vi "OCV Histogram gRPC.vi"() -> (1 "mean values of channels":dbl[](array[numeric]), 2 "std dev":dbl, 3 "range":dbl)   [LabVIEW 2019] (continued)
"battery23voltage"=0.0, "battery24voltage"=0.0, "ErrorOutData"={"ErrorCode"=0, "ErrorMessage"=""}}, {"battery1voltage"=3.48165, "battery2voltage"=3.4830537, "battery3voltage"=3.478374, "battery4voltage"=3.482381, "battery5voltage"=3.4844167, "battery6voltage"=0.0, "battery7voltage"=0.0, "battery8voltage"=0.0, "battery9voltage"=0.0, "battery10voltage"=0.0, "battery11voltage"=0.0, "battery12voltage"=0.0, "battery13voltage"=0.0, "battery14voltage"=0.0, "battery15voltage"=0.0, "battery16voltage"=0.0, "battery17voltage"=0.0, "battery18voltage"=0.0, "battery19voltage"=0.0, "battery20voltage"=0.0, "battery21voltage"=0.0, "battery22voltage"=0.0, "battery23voltage"=0.0, "battery24voltage"=0.0, "ErrorOutData"={"ErrorCode"=0, "ErrorMessage"=""}}, {"battery1voltage"=3.4816468, "battery2voltage"=3.4830554, "battery3voltage"=3.478373, "battery4voltage"=3.482378, "battery5voltage"=3.4844193, "battery6voltage"=0.0, "battery7voltage"=0.0, "battery8voltage"=0.0, "battery9voltage"=0.0, "battery10voltage"=0.0, "battery11voltage"=0.0, "battery12voltage"=0.0, "battery13voltage"=0.0, "battery14voltage"=0.0, "battery15voltage"=0.0, "battery16voltage"=0.0, "battery17voltage"=0.0, "battery18voltage"=0.0, "battery19voltage"=0.0, "battery20voltage"=0.0, "battery21voltage"=0.0, "battery22voltage"=0.0, "battery23voltage"=0.0, "battery24voltage"=0.0, "ErrorOutData"={"ErrorCode"=0, "ErrorMessage"=""}}, {"battery1voltage"=3.4816458, "battery2voltage"=3.4830527, "battery3voltage"=3.4783716, "battery4voltage"=3.4823792, "battery5voltage"=3.4844203, "battery6voltage"=0.0, "battery7voltage"=0.0, "battery8voltage"=0.0, "battery9voltage"=0.0, "battery10voltage"=0.0, "battery11voltage"=0.0, "battery12voltage"=0.0, "battery13voltage"=0.0, "battery14voltage"=0.0, "battery15voltage"=0.0, "battery16voltage"=0.0, "battery17voltage"=0.0, "battery18voltage"=0.0, "battery19voltage"=0.0, "battery20voltage"=0.0, "battery21voltage"=0.0, "battery22voltage"=0.0, "battery23voltage"=0.0, "battery24voltage"=0.0, "ErrorOutData"={"ErrorCode"=0, "ErrorMessage"=""}}, {"battery1voltage"=3.4816468, "battery2voltage"=3.4830546, "battery3voltage"=3.4783747, "battery4voltage"=3.4823809, "battery5voltage"=3.4844174, "battery6voltage"=0.0, "battery7voltage"=0.0, "battery8voltage"=0.0, "battery9voltage"=0.0, "battery10voltage"=0.0, "battery11voltage"=0.0, "battery12voltage"=0.0, "battery13voltage"=0.0, "battery14voltage"=0.0, "battery15voltage"=0.0, "battery16voltage"=0.0, "battery17voltage"=0.0, "battery18voltage"=0.0, "battery19voltage"=0.0, "battery20voltage"=0.0, "battery21voltage"=0.0, "battery22voltage"=0.0, "battery23voltage"=0.0, "battery24voltage"=0.0, "ErrorOutData"={"ErrorCode"=0, "ErrorMessage"=""}}, {"battery1voltage"=3.4816499, "battery2voltage"=3.483051, "battery3voltage"=3.4783742, "battery4voltage"=3.4823804, "battery5voltage"=3.4844172, "battery6voltage"=0.0, "battery7voltage"=0.0, "battery8voltage"=0.0, "battery9voltage"=0.0, "battery10voltage"=0.0, "battery11voltage"=0.0, "battery12voltage"=0.0, "battery13voltage"=0.0, "battery14voltage"=0.0, "battery15voltage"=0.0, "battery16voltage"=0.0, "battery17voltage"=0.0, "battery18voltage"=0.0, "battery19voltage"=0.0, "battery20voltage"=0.0, "battery21voltage"=0.0, "battery22voltage"=0.0, "battery23voltage"=0.0, "battery24voltage"=0.0, "ErrorOutData"={"ErrorCode"=0, "ErrorMessage"=""}}, {"battery1voltage"=3.481651, "battery2voltage"=3.4830523, "battery3voltage"=3.4783762, "battery4voltage"=3.4823794, "battery5voltage"=3.4844174, "battery6voltage"=0.0, "battery7voltage"=0.0, "battery8voltage"=0.0, "battery9voltage"=0.0, "battery10voltage"=0.0, "battery11voltage"=0.0, "battery12voltage"=0.0, "battery13voltage"=0.0, "battery14voltage"=0.0, "battery15voltage"=0.0, "battery16voltage"=0.0, "battery17voltage"=0.0, "battery18voltage"=0.0, "battery19voltage"=0.0, "battery20voltage"=0.0, "battery21voltage"=0.0, "battery22voltage"=0.0, "battery23voltage"=0.0, "battery24voltage"=0.0, "ErrorOutData"={"ErrorCode"=0, "ErrorMessage"=""}}, {"battery1voltage"=3.4816477, "battery2voltage"=3.4830496, "battery3voltage"=3.4783719, "battery4voltage"=3.4823775, "battery5voltage"=3.484423, "battery6voltage"=0.0, "battery7voltage"=0.0, "battery8voltage"=0.0, "battery9voltage"=0.0, "battery10voltage"=0.0, "battery11voltage"=0.0, "battery12voltage"=0.0, "battery13voltage"=0.0, "battery14voltage"=0.0, "battery15voltage"=0.0, "battery16voltage"=0.0, "battery17voltage"=0.0, "battery18voltage"=0.0, "battery19voltage"=0.0, "battery20voltage"=0.0, "battery21voltage"=0.0, "battery22voltage"=0.0, "battery23voltage"=0.0, "battery24voltage"=0.0, "ErrorOutData"={"ErrorCode"=0, "ErrorMessage"=""}}, {"battery1voltage"=3.481648, "battery2voltage"=3.4830532, "battery3voltage"=3.4783773, "battery4voltage"=3.4823756, "battery5voltage"=3.4844205, "battery6voltage"=0.0, "battery7voltage"=0.0, "battery8voltage"=0.0, "battery9voltage"=0.0, "battery10voltage"=0.0, "battery11voltage"=0.0, "battery12voltage"=0.0, "battery13voltage"=0.0, "battery14voltage"=0.0, "battery15voltage"=0.0, "battery16voltage"=0.0, "battery17voltage"=0.0, "battery18voltage"=0.0, "battery19voltage"=0.0, "battery20voltage"=0.0, "battery21voltage"=0.0, "battery22voltage"=0.0, "battery23voltage"=0.0, "battery24voltage"=0.0, "ErrorOutData"={"ErrorCode"=0, "ErrorMessage"=""}}, {"battery1voltage"=3.48165, "battery2voltage"=3.483056, "battery3voltage"=3.4783745, "battery4voltage"=3.4823809, "battery5voltage"=3.484417, "battery6voltage"=0.0, "battery7voltage"=0.0, "battery8voltage"=0.0, "battery9voltage"=0.0, "battery10voltage"=0.0, "battery11voltage"=0.0, "battery12voltage"=0.0, "battery13voltage"=0.0, "battery14voltage"=0.0, "battery15voltage"=0.0, "battery16voltage"=0.0, "battery17voltage"=0.0, "battery18voltage"=0.0, "battery19voltage"=0.0, "battery20voltage"=0.0, "battery21voltage"=0.0, "battery22voltage"=0.0, "battery23voltage"=0.0, "battery24voltage"=0.0, "ErrorOutData"={"ErrorCode"=0, "ErrorMessage"=""}}, {"battery1voltage"=3.481646, "battery2voltage"=3.4830534, "battery3voltage"=3.4783778, "battery4voltage"=3.482377, "battery5voltage"=3.4844174, "battery6voltage"=0.0, "battery7voltage"=0.0, "battery8voltage"=0.0, "battery9voltage"=0.0, "battery10voltage"=0.0, "battery11voltage"=0.0, "battery12voltage"=0.0, "battery13voltage"=0.0, "battery14voltage"=0.0, "battery15voltage"=0.0, "battery16voltage"=0.0, "battery17voltage"=0.0, "battery18voltage"=0.0, "battery19voltage"=0.0, "battery20voltage"=0.0, "battery21voltage"=0.0, "battery22voltage"=0.0, "battery23voltage"=0.0, "battery24voltage"=0.0, "ErrorOutData"={"ErrorCode"=0, "ErrorMessage"=""}}, {"battery1voltage"=3.4816492, "battery2voltage"=3.483059, "battery3voltage"=3.4783738, "battery4voltage"=3.4823813, "battery5voltage"=3.4844182, "battery6voltage"=0.0, "battery7voltage"=0.0, "battery8voltage"=0.0, "battery9voltage"=0.0, "battery10voltage"=0.0, "battery11voltage"=0.0, "battery12voltage"=0.0, "battery13voltage"=0.0, "battery14voltage"=0.0, "battery15voltage"=0.0, "battery16voltage"=0.0, "battery17voltage"=0.0, "battery18voltage"=0.0, "battery19voltage"=0.0, "battery20voltage"=0.0, "battery21voltage"=0.0, "battery22voltage"=0.0, "battery23voltage"=0.0, "battery24voltage"=0.0, "ErrorOutData"={"ErrorCode"=0, "ErrorMessage"=""}}, {"battery1voltage"=3.4816453, "battery2voltage"=3.483056, "battery3voltage"=3.4783773, "battery4voltage"=3.48238, "battery5voltage"=3.4844167, "battery6voltage"=0.0, "battery7voltage"=0.0, "battery8voltage"=0.0, "battery9voltage"=0.0, "battery10voltage"=0.0, "battery11voltage"=0.0, "battery12voltage"=0.0, "battery13voltage"=0.0, "battery14voltage"=0.0, "battery15voltage"=0.0, "battery16voltage"=0.0, "battery17voltage"=0.0, "battery18voltage"=0.0, "battery19voltage"=0.0, "battery20voltage"=0.0, "battery21voltage"=0.0, "battery22voltage"=0.0, "battery23voltage"=0.0, "battery24voltage"=0.0, "ErrorOutData"={"ErrorCode"=0, "ErrorMessage"=""}}, {"battery1voltage"=3.4816477, "battery2voltage"=3.4830568, "battery3voltage"=3.478376, "battery4voltage"=3.4823825, "battery5voltage"=3.4844162, "battery6voltage"=0.0, "battery7voltage"=0.0, "battery8voltage"=0.0, "battery9voltage"=0.0, "battery10voltage"=0.0, "battery11voltage"=0.0, "battery12voltage"=0.0, "battery13voltage"=0.0, "battery14voltage"=0.0, "battery15voltage"=0.0, "battery16voltage"=0.0, "battery17voltage"=0.0, "battery18voltage"=0.0, "battery19voltage"=0.0, "battery20voltage"=0.0, "battery21voltage"=0.0, "battery22voltage"=0.0, "battery23voltage"=0.0, "battery24voltage"=0.0, "ErrorOutData"={"ErrorCode"=0, "ErrorMessage"=""}}, {"battery1voltage"=3.4816475, "battery2voltage"=3.4830549, "battery3voltage"=3.4783726, "battery4voltage"=3.4823778, "battery5voltage"=3.4844217, "battery6voltage"=0.0, "battery7voltage"=0.0, "battery8voltage"=0.0, "battery9voltage"=0.0, "battery10voltage"=0.0, "battery11voltage"=0.0, "battery12voltage"=0.0, "battery13voltage"=0.0, "battery14voltage"=0.0, "battery15voltage"=0.0, "battery16voltage"=0.0, "battery17voltage"=0.0, "battery18voltage"=0.0, "battery19voltage"=0.0, "battery20voltage"=0.0, "battery21voltage"=0.0, "battery22voltage"=0.0, "battery23voltage"=0.0, "battery24voltage"=0.0, "ErrorOutData"={"ErrorCode"=0, "ErrorMessage"=""}}, {"battery1voltage"=3.481645, "battery2voltage"=3.4830534, "battery3voltage"=3.4783769, "battery4voltage"=3.4823775, "battery5voltage"=3.4844167, "battery6voltage"=0.0, "battery7voltage"=0.0, "battery8voltage"=0.0, "battery9voltage"=0.0, "battery10voltage"=0.0, "battery11voltage"=0.0, "battery12voltage"=0.0, "battery13voltage"=0.0, "battery14voltage"=0.0, "battery15voltage"=0.0, "battery16voltage"=0.0, "battery17voltage"=0.0, "battery18voltage"=0.0, "battery19voltage"=0.0, "battery20voltage"=0.0, "battery21voltage"=0.0, "battery22voltage"=0.0, "battery23voltage"=0.0, "battery24voltage"=0.0, "ErrorOutData"={"ErrorCode"=0, "ErrorMessage"=""}}, {"battery1voltage"=3.4816496, "battery2voltage"=3.4830532, "battery3voltage"=3.4783723, "battery4voltage"=3.4823792, "battery5voltage"=3.4844182, "battery6voltage"=0.0, "battery7voltage"=0.0, "battery8voltage"=0.0, "battery9voltage"=0.0, "battery10voltage"=0.0, "battery11voltage"=0.0, "battery12voltage"=0.0, "battery13voltage"=0.0, "battery14voltage"=0.0, "battery15voltage"=0.0, "battery16voltage"=0.0, "battery17voltage"=0.0, "battery18voltage"=0.0, "battery19voltage"=0.0, "battery20voltage"=0.0, "battery21voltage"=0.0, "battery22voltage"=0.0, "battery23voltage"=0.0, "battery24voltage"=0.0, "ErrorOutData"={"ErrorCode"=0, "ErrorMessage"=""}}, {"battery1voltage"=3.481645, "battery2voltage"=3.4830527, "battery3voltage"=3.4783733, "battery4voltage"=3.4823792, "battery5voltage"=3.4844215, "battery6voltage"=0.0, "battery7voltage"=0.0, "battery8voltage"=0.0, "battery9voltage"=0.0, "battery10voltage"=0.0, "battery11voltage"=0.0, "battery12voltage"=0.0, "battery13voltage"=0.0, "battery14voltage"=0.0, "battery15voltage"=0.0, "battery16voltage"=0.0, "battery17voltage"=0.0, "battery18voltage"=0.0, "battery19voltage"=0.0, "battery20voltage"=0.0, "battery21voltage"=0.0, "battery22voltage"=0.0, "battery23voltage"=0.0, "battery24voltage"=0.0, "ErrorOutData"={"ErrorCode"=0, "ErrorMessage"=""}}, {"battery1voltage"=3.4816506, "battery2voltage"=3.4830568, "battery3voltage"=3.4783769, "battery4voltage"=3.4823804, "battery5voltage"=3.484417, "battery6voltage"=0.0, "battery7voltage"=0.0, "battery8voltage"=0.0, "battery9voltage"=0.0, "battery10voltage"=0.0, "battery11voltage"=0.0, "battery12voltage"=0.0, "battery13voltage"=0.0, "battery14voltage"=0.0, "battery15voltage"=0.0, "battery16voltage"=0.0, "battery17voltage"=0.0, "battery18voltage"=0.0, "battery19voltage"=0.0, "battery20voltage"=0.0, "battery21voltage"=0.0, "battery22voltage"=0.0, "battery23voltage"=0.0, "battery24voltage"=0.0, "ErrorOutData"={"ErrorCode"=0, "ErrorMessage"=""}}, {"battery1voltage"=3.4816432, "battery2voltage"=3.483051, "battery3voltage"=3.4783752, "battery4voltage"=3.482378, "battery5voltage"=3.4844196, "battery6voltage"=0.0, "battery7voltage"=0.0, "battery8voltage"=0.0, "battery9voltage"=0.0, "battery10voltage"=0.0, "battery11voltage"=0.0, "battery12voltage"=0.0, "battery13voltage"=0.0, "battery14voltage"=0.0, "battery15voltage"=0.0, "battery16voltage"=0.0, "battery17voltage"=0.0, "battery18voltage"=0.0, "battery19voltage"=0.0, "battery20voltage"=0.0, "battery21voltage"=0.0, "battery22voltage"=0.0, "battery23voltage"=0.0, "battery24voltage"=0.0, "ErrorOutData"={"ErrorCode"=0, "ErrorMessage"=""}}, {"battery1voltage"=3.4816463, "battery2voltage"=3.4830475, "battery3voltage"=3.478373, "battery4voltage"=3.4823802, "battery5voltage"=3.4844208, "battery6voltage"=0.0, "battery7voltage"=0.0, "battery8voltage"=0.0, "battery9voltage"=0.0, "battery10voltage"=0.0, "battery11voltage"=0.0, "battery12voltage"=0.0, "battery13voltage"=0.0, "battery14voltage"=0.0, "battery15voltage"=0.0, "battery16voltage"=0.0, "battery17voltage"=0.0, "battery18voltage"=0.0, "battery19voltage"=0.0, "battery20voltage"=0.0, "battery21voltage"=0.0, "battery22voltage"=0.0, "battery23voltage"=0.0, "battery24voltage"=0.0, "ErrorOutData"={"ErrorCode"=0, "ErrorMessage"=""}}, {"battery1voltage"=3.4816473, "battery2voltage"=3.4830577, "battery3voltage"=3.4783766, "battery4voltage"=3.4823806, "battery5voltage"=3.484416, "battery6voltage"=0.0, "battery7voltage"=0.0, "battery8voltage"=0.0, "battery9voltage"=0.0, "battery10voltage"=0.0, "battery11voltage"=0.0, "battery12voltage"=0.0, "battery13voltage"=0.0, "battery14voltage"=0.0, "battery15voltage"=0.0, "battery16voltage"=0.0, "battery17voltage"=0.0, "battery18voltage"=0.0, "battery19voltage"=0.0, "battery20voltage"=0.0, "battery21voltage"=0.0, "battery22voltage"=0.0, "battery23voltage"=0.0, "battery24voltage"=0.0, "ErrorOutData"={"ErrorCode"=0, "ErrorMessage"=""}}, {"battery1voltage"=3.4816453, "battery2voltage"=3.4830537, "battery3voltage"=3.478374, "battery4voltage"=3.48238, "battery5voltage"=3.4844222, "battery6voltage"=0.0, "battery7voltage"=0.0, "battery8voltage"=0.0, "battery9voltage"=0.0, "battery10voltage"=0.0, "battery11voltage"=0.0, "battery12voltage"=0.0, "battery13voltage"=0.0, "battery14voltage"=0.0, "battery15voltage"=0.0, "battery16voltage"=0.0, "battery17voltage"=0.0, "battery18voltage"=0.0, "battery19voltage"=0.0, "battery20voltage"=0.0, "battery21voltage"=0.0, "battery22voltage"=0.0, "battery23voltage"=0.0, "battery24voltage"=0.0, "ErrorOutData"={"ErrorCode"=0, "ErrorMessage"=""}}, {"battery1voltage"=3.4816496, "battery2voltage"=3.4830496, "battery3voltage"=3.4783752, "battery4voltage"=3.4823782, "battery5voltage"=3.4844208, "battery6voltage"=0.0, "battery7voltage"=0.0, "battery8voltage"=0.0, "battery9voltage"=0.0, "battery10voltage"=0.0, "battery11voltage"=0.0, "battery12voltage"=0.0, "battery13voltage"=0.0, "battery14voltage"=0.0, "battery15voltage"=0.0, "battery16voltage"=0.0, "battery17voltage"=0.0, "battery18voltage"=0.0, "battery19voltage"=0.0, "battery20voltage"=0.0, "battery21voltage"=0.0, "battery22voltage"=0.0, "battery23voltage"=0.0, "battery24voltage"=0.0, "ErrorOutData"={"ErrorCode"=0, "ErrorMessage"=""}}, {"battery1voltage"=3.481648, "battery2voltage"=3.483055, "battery3voltage"=3.4783757, "battery4voltage"=3.4823782, "battery5voltage"=3.484418, "battery6voltage"=0.0, "battery7voltage"=0.0, "battery8voltage"=0.0, "battery9voltage"=0.0, "battery10voltage"=0.0, "battery11voltage"=0.0, "battery12voltage"=0.0, "battery13voltage"=0.0, "battery14voltage"=0.0, "battery15voltage"=0.0, "battery16voltage"=0.0, "battery17voltage"=0.0, "battery18voltage"=0.0, "battery19voltage"=0.0, "battery20voltage"=0.0, "battery21voltage"=0.0, "battery22voltage"=0.0, "battery23voltage"=0.0, "battery24voltage"=0.0, "ErrorOutData"={"ErrorCode"=0, "ErrorMessage"=""}}, {"battery1voltage"=3.4816477, "battery2voltage"=3.4830513, "battery3voltage"=3.4783764, "battery4voltage"=3.4823806, "battery5voltage"=3.4844177, "battery6voltage"=0.0, "battery7voltage"=0.0, "battery8voltage"=0.0, "battery9voltage"=0.0, "battery10voltage"=0.0, "battery11voltage"=0.0, "battery12voltage"=0.0, "battery13voltage"=0.0, "battery14voltage"=0.0, "battery15voltage"=0.0, "battery16voltage"=0.0, "battery17voltage"=0.0, "battery18voltage"=0.0, "battery19voltage"=0.0, "battery20voltage"=0.0, "battery21voltage"=0.0, "battery22voltage"=0.0, "battery23voltage"=0.0, "battery24voltage"=0.0, "ErrorOutData"={"ErrorCode"=0, "ErrorMessage"=""}}, {"battery1voltage"=3.4816487, "battery2voltage"=3.4830525, "battery3voltage"=3.4783738, "battery4voltage"=3.4823785, "battery5voltage"=3.4844203, "battery6voltage"=0.0, "battery7voltage"=0.0, "battery8voltage"=0.0, "battery9voltage"=0.0, "battery10voltage"=0.0, "battery11voltage"=0.0, "battery12voltage"=0.0, "battery13voltage"=0.0, "battery14voltage"=0.0, "battery15voltage"=0.0, "battery16voltage"=0.0, "battery17voltage"=0.0, "battery18voltage"=0.0, "battery19voltage"=0.0, "battery20voltage"=0.0, "battery21voltage"=0.0, "battery22voltage"=0.0, "battery23voltage"=0.0, "battery24voltage"=0.0, "ErrorOutData"={"ErrorCode"=0, "ErrorMessage"=""}}, {"battery1voltage"=3.48165, "battery2voltage"=3.4830563, "battery3voltage"=3.4783766, "battery4voltage"=3.4823785, "battery5voltage"=3.484417, "battery6voltage"=0.0, "battery7voltage"=0.0, "battery8voltage"=0.0, "battery9voltage"=0.0, "battery10voltage"=0.0, "battery11voltage"=0.0, "battery12voltage"=0.0, "battery13voltage"=0.0, "battery14voltage"=0.0, "battery15voltage"=0.0, "battery16voltage"=0.0, "battery17voltage"=0.0, "battery18voltage"=0.0, "battery19voltage"=0.0, "battery20voltage"=0.0, "battery21voltage"=0.0, "battery22voltage"=0.0, "battery23voltage"=0.0, "battery24voltage"=0.0, "ErrorOutData"={"ErrorCode"=0, "ErrorMessage"=""}}, {"battery1voltage"=3.4816463, "battery2voltage"=3.4830563, "battery3voltage"=3.478375, "battery4voltage"=3.4823804, "battery5voltage"=3.4844193, "battery6voltage"=0.0, "battery7voltage"=0.0, "battery8voltage"=0.0, "battery9voltage"=0.0, "battery10voltage"=0.0, "battery11voltage"=0.0, "battery12voltage"=0.0, "battery13voltage"=0.0, "battery14voltage"=0.0, "battery15voltage"=0.0, "battery16voltage"=0.0, "battery17voltage"=0.0, "battery18voltage"=0.0, "battery19voltage"=0.0, "battery20voltage"=0.0, "battery21voltage"=0.0, "battery22voltage"=0.0, "battery23voltage"=0.0, "battery24voltage"=0.0, "ErrorOutData"={"ErrorCode"=0, "ErrorMessage"=""}}, {"battery1voltage"=3.481647, "battery2voltage"=3.4830527, "battery3voltage"=3.4783754, "battery4voltage"=3.4823787, "battery5voltage"=3.4844213, "battery6voltage"=0.0, "battery7voltage"=0.0, "battery8voltage"=0.0, "battery9voltage"=0.0, "battery10voltage"=0.0, "battery11voltage"=0.0, "battery12voltage"=0.0, "battery13voltage"=0.0, "battery14voltage"=0.0, "battery15voltage"=0.0, "battery16voltage"=0.0, "battery17voltage"=0.0, "battery18voltage"=0.0, "battery19voltage"=0.0, "battery20voltage"=0.0, "battery21voltage"=0.0, "battery22voltage"=0.0, "battery23voltage"=0.0, "battery24voltage"=0.0, "ErrorOutData"={"ErrorCode"=0, "ErrorMessage"=""}}, {"battery1voltage"=3.4816496, "battery2voltage"=3.4830544, "battery3voltage"=3.4783766, "battery4voltage"=3.4823828, "battery5voltage"=3.4844184, "battery6voltage"=0.0, "battery7voltage"=0.0, "battery8voltage"=0.0, "battery9voltage"=0.0, "battery10voltage"=0.0, "battery11voltage"=0.0, "battery12voltage"=0.0, "battery13voltage"=0.0, "battery14voltage"=0.0, "battery15voltage"=0.0, "battery16voltage"=0.0, "battery17voltage"=0.0, "battery18voltage"=0.0, "battery19voltage"=0.0, "battery20voltage"=0.0, "battery21voltage"=0.0, "battery22voltage"=0.0, "battery23voltage"=0.0, "battery24voltage"=0.0, "ErrorOutData"={"ErrorCode"=0, "ErrorMessage"=""}}, {"battery1voltage"=3.48165, "battery2voltage"=3.4830563, "battery3voltage"=3.4783742, "battery4voltage"=3.4823813, "battery5voltage"=3.4844193, "battery6voltage"=0.0, "battery7voltage"=0.0, "battery8voltage"=0.0, "battery9voltage"=0.0, "battery10voltage"=0.0, "battery11voltage"=0.0, "battery12voltage"=0.0, "battery13voltage"=0.0, "battery14voltage"=0.0, "battery15voltage"=0.0, "battery16voltage"=0.0, "battery17voltage"=0.0, "battery18voltage"=0.0, "battery19voltage"=0.0, "battery20voltage"=0.0, "battery21voltage"=0.0, "battery22voltage"=0.0, "battery23voltage"=0.0, "battery24voltage"=0.0, "ErrorOutData"={"ErrorCode"=0, "ErrorMessage"=""}}, {"battery1voltage"=3.4816482, "battery2voltage"=3.4830506, "battery3voltage"=3.4783733, "battery4voltage"=3.482379, "battery5voltage"=3.4844246, "battery6voltage"=0.0, "battery7voltage"=0.0, "battery8voltage"=0.0, "battery9voltage"=0.0, "battery10voltage"=0.0, "battery11voltage"=0.0, "battery12voltage"=0.0, "battery13voltage"=0.0, "battery14voltage"=0.0, "battery15voltage"=0.0, "battery16voltage"=0.0, "battery17voltage"=0.0, "battery18voltage"=0.0, "battery19voltage"=0.0, "battery20voltage"=0.0, "battery21voltage"=0.0, "battery22voltage"=0.0, "battery23voltage"=0.0, "battery24voltage"=0.0, "ErrorOutData"={"ErrorCode"=0, "ErrorMessage"=""}}, {"battery1voltage"=3.481647, "battery2voltage"=3.48305, "battery3voltage"=3.47837, "battery4voltage"=3.4823792, "battery5voltage"=3.4844222, "battery6voltage"=0.0, "battery7voltage"=0.0, "battery8voltage"=0.0, "battery9voltage"=0.0, "battery10voltage"=0.0, "battery11voltage"=0.0, "battery12voltage"=0.0, "battery13voltage"=0.0, "battery14voltage"=0.0, "battery15voltage"=0.0, "battery16voltage"=0.0, "battery17voltage"=0.0, "battery18voltage"=0.0, "battery19voltage"=0.0, "battery20voltage"=0.0, "battery21voltage"=0.0, "battery22voltage"=0.0, "battery23voltage"=0.0, "battery24voltage"=0.0, "ErrorOutData"={"ErrorCode"=0, "ErrorMessage"=""}}, {"battery1voltage"=3.4816499, "battery2voltage"=3.4830544, "battery3voltage"=3.478378, "battery4voltage"=3.4823816, "battery5voltage"=3.4844143, "battery6voltage"=0.0, "battery7voltage"=0.0, "battery8voltage"=0.0, "battery9voltage"=0.0, "battery10voltage"=0.0, "battery11voltage"=0.0, "battery12voltage"=0.0, "battery13voltage"=0.0, "battery14voltage"=0.0, "battery15voltage"=0.0, "battery16voltage"=0.0, "battery17voltage"=0.0, "battery18voltage"=0.0, "battery19voltage"=0.0, "battery20voltage"=0.0, "battery21voltage"=0.0, "battery22voltage"=0.0, "battery23voltage"=0.0, "battery24voltage"=0.0, "ErrorOutData"={"ErrorCode"=0, "ErrorMessage"=""}}, {"battery1voltage"=3.4816465, "battery2voltage"=3.4830492, "battery3voltage"=3.4783719, "battery4voltage"=3.4823792, "battery5voltage"=3.4844215, "battery6voltage"=0.0, "battery7voltage"=0.0, "battery8voltage"=0.0, "battery9voltage"=0.0, "battery10voltage"=0.0, "battery11voltage"=0.0, "battery12voltage"=0.0, "battery13voltage"=0.0, "battery14voltage"=0.0, "battery15voltage"=0.0, "battery16voltage"=0.0, "battery17voltage"=0.0, "battery18voltage"=0.0, "battery19voltage"=0.0, "battery20voltage"=0.0, "battery21voltage"=0.0, "battery22voltage"=0.0, "battery23voltage"=0.0, "battery24voltage"=0.0, "ErrorOutData"={"ErrorCode"=0, "ErrorMessage"=""}}, {"battery1voltage"=3.481645, "battery2voltage"=3.4830499, "battery3voltage"=3.4783711, "battery4voltage"=3.4823794, "battery5voltage"=3.4844224, "battery6voltage"=0.0, "battery7voltage"=0.0, "battery8voltage"=0.0, "battery9voltage"=0.0, "battery10voltage"=0.0, "battery11voltage"=0.0, "battery12voltage"=0.0, "battery13voltage"=0.0, "battery14voltage"=0.0, "battery15voltage"=0.0, "battery16voltage"=0.0, "battery17voltage"=0.0, "battery18voltage"=0.0, "battery19voltage"=0.0, "battery20voltage"=0.0, "battery21voltage"=0.0, "battery22voltage"=0.0, "battery23voltage"=0.0, "battery24voltage"=0.0, "ErrorOutData"={"ErrorCode"=0, "ErrorMessage"=""}}, {"battery1voltage"=3.481649, "battery2voltage"=3.4830532, "battery3voltage"=3.4783745, "battery4voltage"=3.4823806, "battery5voltage"=3.4844162, "battery6voltage"=0.0, "battery7voltage"=0.0, "battery8voltage"=0.0, "battery9voltage"=0.0, "battery10voltage"=0.0, "battery11voltage"=0.0, "battery12voltage"=0.0, "battery13voltage"=0.0, "battery14voltage"=0.0, "battery15voltage"=0.0, "battery16voltage"=0.0, "battery17voltage"=0.0, "battery18voltage"=0.0, "battery19voltage"=0.0, "battery20voltage"=0.0, "battery21voltage"=0.0, "battery22voltage"=0.0, "battery23voltage"=0.0, "battery24voltage"=0.0, "ErrorOutData"={"ErrorCode"=0, "ErrorMessage"=""}}, {"battery1voltage"=3.4816484, "battery2voltage"=3.4830568, "battery3voltage"=3.4783745, "battery4voltage"=3.4823828, "battery5voltage"=3.4844155, "battery6voltage"=0.0, "battery7voltage"=0.0, "battery8voltage"=0.0, "battery9voltage"=0.0, "battery10voltage"=0.0, "battery11voltage"=0.0, "battery12voltage"=0.0, "battery13voltage"=0.0, "battery14voltage"=0.0, "battery15voltage"=0.0, "battery16voltage"=0.0, "battery17voltage"=0.0, "battery18voltage"=0.0, "battery19voltage"=0.0, "battery20voltage"=0.0, "battery21voltage"=0.0, "battery22voltage"=0.0, "battery23voltage"=0.0, "battery24voltage"=0.0, "ErrorOutData"={"ErrorCode"=0, "ErrorMessage"=""}}, {"battery1voltage"=3.4816473, "battery2voltage"=3.4830527, "battery3voltage"=3.4783683, "battery4voltage"=3.482379, "battery5voltage"=3.4844186, "battery6voltage"=0.0, "battery7voltage"=0.0, "battery8voltage"=0.0, "battery9voltage"=0.0, "battery10voltage"=0.0, "battery11voltage"=0.0, "battery12voltage"=0.0, "battery13voltage"=0.0, "battery14voltage"=0.0, "battery15voltage"=0.0, "battery16voltage"=0.0, "battery17voltage"=0.0, "battery18voltage"=0.0, "battery19voltage"=0.0, "battery20voltage"=0.0, "battery21voltage"=0.0, "battery22voltage"=0.0, "battery23voltage"=0.0, "battery24voltage"=0.0, "ErrorOutData"={"ErrorCode"=0, "ErrorMessage"=""}}, {"battery1voltage"=3.481651, "battery2voltage"=3.4830503, "battery3voltage"=3.478369, "battery4voltage"=3.482383, "battery5voltage"=3.4844155, "battery6voltage"=0.0, "battery7voltage"=0.0, "battery8voltage"=0.0, "battery9voltage"=0.0, "battery10voltage"=0.0, "battery11voltage"=0.0, "battery12voltage"=0.0, "battery13voltage"=0.0, "battery14voltage"=0.0, "battery15voltage"=0.0, "battery16voltage"=0.0, "battery17voltage"=0.0, "battery18voltage"=0.0, "battery19voltage"=0.0, "battery20voltage"=0.0, "battery21voltage"=0.0, "battery22voltage"=0.0, "battery23voltage"=0.0, "battery24voltage"=0.0, "ErrorOutData"={"ErrorCode"=0, "ErrorMessage"=""}}, {"battery1voltage"=3.4816494, "battery2voltage"=3.48305, "battery3voltage"=3.4783678, "battery4voltage"=3.4823797, "battery5voltage"=3.4844215, "battery6voltage"=0.0, "battery7voltage"=0.0, "battery8voltage"=0.0, "battery9voltage"=0.0, "battery10voltage"=0.0, "battery11voltage"=0.0, "battery12voltage"=0.0, "battery13voltage"=0.0, "battery14voltage"=0.0, "battery15voltage"=0.0, "battery16voltage"=0.0, "battery17voltage"=0.0, "battery18voltage"=0.0, "battery19voltage"=0.0, "battery20voltage"=0.0, "battery21voltage"=0.0, "battery22voltage"=0.0, "battery23voltage"=0.0, "battery24voltage"=0.0, "ErrorOutData"={"ErrorCode"=0, "ErrorMessage"=""}}, {"battery1voltage"=3.4816449, "battery2voltage"=3.4830515, "battery3voltage"=3.4783702, "battery4voltage"=3.4823787, "battery5voltage"=3.4844258, "battery6voltage"=0.0, "battery7voltage"=0.0, "battery8voltage"=0.0, "battery9voltage"=0.0, "battery10voltage"=0.0, "battery11voltage"=0.0, "battery12voltage"=0.0, "battery13voltage"=0.0, "battery14voltage"=0.0, "battery15voltage"=0.0, "battery16voltage"=0.0, "battery17voltage"=0.0, "battery18voltage"=0.0, "battery19voltage"=0.0, "battery20voltage"=0.0, "battery21voltage"=0.0, "battery22voltage"=0.0, "battery23voltage"=0.0, "battery24voltage"=0.0, "ErrorOutData"={"ErrorCode"=0, "ErrorMessage"=""}}, {"battery1voltage"=3.4816527, "battery2voltage"=3.4830549, "battery3voltage"=3.4783728, "battery4voltage"=3.4823782, "battery5voltage"=3.484418, "battery6voltage"=0.0, "battery7voltage"=0.0, "battery8voltage"=0.0, "battery9voltage"=0.0, "battery10voltage"=0.0, "battery11voltage"=0.0, "battery12voltage"=0.0, "battery13voltage"=0.0, "battery14voltage"=0.0, "battery15voltage"=0.0, "battery16voltage"=0.0, "battery17voltage"=0.0, "battery18voltage"=0.0, "battery19voltage"=0.0, "battery20voltage"=0.0, "battery21voltage"=0.0, "battery22voltage"=0.0, "battery23voltage"=0.0, "battery24voltage"=0.0, "ErrorOutData"={"ErrorCode"=0, "ErrorMessage"=""}}, {"battery1voltage"=3.4816496, "battery2voltage"=3.4830508, "battery3voltage"=3.478367, "battery4voltage"=3.4823806, "battery5voltage"=3.4844215, "battery6voltage"=0.0, "battery7voltage"=0.0, "battery8voltage"=0.0, "battery9voltage"=0.0, "battery10voltage"=0.0, "battery11voltage"=0.0, "battery12voltage"=0.0, "battery13voltage"=0.0, "battery14voltage"=0.0, "battery15voltage"=0.0, "battery16voltage"=0.0, "battery17voltage"=0.0, "battery18voltage"=0.0, "battery19voltage"=0.0, "battery20voltage"=0.0, "battery21voltage"=0.0, "battery22voltage"=0.0, "battery23voltage"=0.0, "battery24voltage"=0.0, "ErrorOutData"={"ErrorCode"=0, "ErrorMessage"=""}}, {"battery1voltage"=3.4816458, "battery2voltage"=3.4830508, "battery3voltage"=3.478366, "battery4voltage"=3.4823809, "battery5voltage"=3.4844244, "battery6voltage"=0.0, "battery7voltage"=0.0, "battery8voltage"=0.0, "battery9voltage"=0.0, "battery10voltage"=0.0, "battery11voltage"=0.0, "battery12voltage"=0.0, "battery13voltage"=0.0, "battery14voltage"=0.0, "battery15voltage"=0.0, "battery16voltage"=0.0, "battery17voltage"=0.0, "battery18voltage"=0.0, "battery19voltage"=0.0, "battery20voltage"=0.0, "battery21voltage"=0.0, "battery22voltage"=0.0, "battery23voltage"=0.0, "battery24voltage"=0.0, "ErrorOutData"={"ErrorCode"=0, "ErrorMessage"=""}}, {"battery1voltage"=3.4816482, "battery2voltage"=3.4830556, "battery3voltage"=3.4783711, "battery4voltage"=3.482381, "battery5voltage"=3.484418, "battery6voltage"=0.0, "battery7voltage"=0.0, "battery8voltage"=0.0, "battery9voltage"=0.0, "battery10voltage"=0.0, "battery11voltage"=0.0, "battery12voltage"=0.0, "battery13voltage"=0.0, "battery14voltage"=0.0, "battery15voltage"=0.0, "battery16voltage"=0.0, "battery17voltage"=0.0, "battery18voltage"=0.0, "battery19voltage"=0.0, "battery20voltage"=0.0, "battery21voltage"=0.0, "battery22voltage"=0.0, "battery23voltage"=0.0, "battery24voltage"=0.0, "ErrorOutData"={"ErrorCode"=0, "ErrorMessage"=""}}, {"battery1voltage"=3.4816434, "battery2voltage"=3.4830503, "battery3voltage"=3.4783661, "battery4voltage"=3.4823787, "battery5voltage"=3.4844215, "battery6voltage"=0.0, "battery7voltage"=0.0, "battery8voltage"=0.0, "battery9voltage"=0.0, "battery10voltage"=0.0, "battery11voltage"=0.0, "battery12voltage"=0.0, "battery13voltage"=0.0, "battery14voltage"=0.0, "battery15voltage"=0.0, "battery16voltage"=0.0, "battery17voltage"=0.0, "battery18voltage"=0.0, "battery19voltage"=0.0, "battery20voltage"=0.0, "battery21voltage"=0.0, "battery22voltage"=0.0, "battery23voltage"=0.0, "battery24voltage"=0.0, "ErrorOutData"={"ErrorCode"=0, "ErrorMessage"=""}}, {"battery1voltage"=3.4816463, "battery2voltage"=3.483053, "battery3voltage"=3.4783685, "battery4voltage"=3.4823806, "battery5voltage"=3.484423, "battery6voltage"=0.0, "battery7voltage"=0.0, "battery8voltage"=0.0, "battery9voltage"=0.0, "battery10voltage"=0.0, "battery11voltage"=0.0, "battery12voltage"=0.0, "battery13voltage"=0.0, "battery14voltage"=0.0, "battery15voltage"=0.0, "battery16voltage"=0.0, "battery17voltage"=0.0, "battery18voltage"=0.0, "battery19voltage"=0.0, "battery20voltage"=0.0, "battery21voltage"=0.0, "battery22voltage"=0.0, "battery23voltage"=0.0, "battery24voltage"=0.0, "ErrorOutData"={"ErrorCode"=0, "ErrorMessage"=""}}, {"battery1voltage"=3.4816482, "battery2voltage"=3.4830568, "battery3voltage"=3.4783738, "battery4voltage"=3.4823809, "battery5voltage"=3.4844167, "battery6voltage"=0.0, "battery7voltage"=0.0, "battery8voltage"=0.0, "battery9voltage"=0.0, "battery10voltage"=0.0, "battery11voltage"=0.0, "battery12voltage"=0.0, "battery13voltage"=0.0, "battery14voltage"=0.0, "battery15voltage"=0.0, "battery16voltage"=0.0, "battery17voltage"=0.0, "battery18voltage"=0.0, "battery19voltage"=0.0, "battery20voltage"=0.0, "battery21voltage"=0.0, "battery22voltage"=0.0, "battery23voltage"=0.0, "battery24voltage"=0.0, "ErrorOutData"={"ErrorCode"=0, "ErrorMessage"=""}}, {"battery1voltage"=3.4816475, "battery2voltage"=3.4830494, "battery3voltage"=3.4783683, "battery4voltage"=3.4823792, "battery5voltage"=3.48442, "battery6voltage"=0.0, "battery7voltage"=0.0, "battery8voltage"=0.0, "battery9voltage"=0.0, "battery10voltage"=0.0, "battery11voltage"=0.0, "battery12voltage"=0.0, "battery13voltage"=0.0, "battery14voltage"=0.0, "battery15voltage"=0.0, "battery16voltage"=0.0, "battery17voltage"=0.0, "battery18voltage"=0.0, "battery19voltage"=0.0, "battery20voltage"=0.0, "battery21voltage"=0.0, "battery22voltage"=0.0, "battery23voltage"=0.0, "battery24voltage"=0.0, "ErrorOutData"={"ErrorCode"=0, "ErrorMessage"=""}}, {"battery1voltage"=3.4816458, "battery2voltage"=3.4830513, "battery3voltage"=3.4783676, "battery4voltage"=3.4823787, "battery5voltage"=3.4844215, "battery6voltage"=0.0, "battery7voltage"=0.0, "battery8voltage"=0.0, "battery9voltage"=0.0, "battery10voltage"=0.0, "battery11voltage"=0.0, "battery12voltage"=0.0, "battery13voltage"=0.0, "battery14voltage"=0.0, "battery15voltage"=0.0, "battery16voltage"=0.0, "battery17voltage"=0.0, "battery18voltage"=0.0, "battery19voltage"=0.0, "battery20voltage"=0.0, "battery21voltage"=0.0, "battery22voltage"=0.0, "battery23voltage"=0.0, "battery24voltage"=0.0, "ErrorOutData"={"ErrorCode"=0, "ErrorMessage"=""}}, {"battery1voltage"=3.4816453, "battery2voltage"=3.4830549, "battery3voltage"=3.4783688, "battery4voltage"=3.4823809, "battery5voltage"=3.4844248, "battery6voltage"=0.0, "battery7voltage"=0.0, "battery8voltage"=0.0, "battery9voltage"=0.0, "battery10voltage"=0.0, "battery11voltage"=0.0, "battery12voltage"=0.0, "battery13voltage"=0.0, "battery14voltage"=0.0, "battery15voltage"=0.0, "battery16voltage"=0.0, "battery17voltage"=0.0, "battery18voltage"=0.0, "battery19voltage"=0.0, "battery20voltage"=0.0, "battery21voltage"=0.0, "battery22voltage"=0.0, "battery23voltage"=0.0, "battery24voltage"=0.0, "ErrorOutData"={"ErrorCode"=0, "ErrorMessage"=""}}, {"battery1voltage"=3.4816477, "battery2voltage"=3.4830544, "battery3voltage"=3.4783747, "battery4voltage"=3.482379, "battery5voltage"=3.484416, "battery6voltage"=0.0, "battery7voltage"=0.0, "battery8voltage"=0.0, "battery9voltage"=0.0, "battery10voltage"=0.0, "battery11voltage"=0.0, "battery12voltage"=0.0, "battery13voltage"=0.0, "battery14voltage"=0.0, "battery15voltage"=0.0, "battery16voltage"=0.0, "battery17voltage"=0.0, "battery18voltage"=0.0, "battery19voltage"=0.0, "battery20voltage"=0.0, "battery21voltage"=0.0, "battery22voltage"=0.0, "battery23voltage"=0.0, "battery24voltage"=0.0, "ErrorOutData"={"ErrorCode"=0, "ErrorMessage"=""}}, {"battery1voltage"=3.4816506, "battery2voltage"=3.4830523, "battery3voltage"=3.4783723, "battery4voltage"=3.4823835, "battery5voltage"=3.4844174, "battery6voltage"=0.0, "battery7voltage"=0.0, "battery8voltage"=0.0, "battery9voltage"=0.0, "battery10voltage"=0.0, "battery11voltage"=0.0, "battery12voltage"=0.0, "battery13voltage"=0.0, "battery14voltage"=0.0, "battery15voltage"=0.0, "battery16voltage"=0.0, "battery17voltage"=0.0, "battery18voltage"=0.0, "battery19voltage"=0.0, "battery20voltage"=0.0, "battery21voltage"=0.0, "battery22voltage"=0.0, "battery23voltage"=0.0, "battery24voltage"=0.0, "ErrorOutData"={"ErrorCode"=0, "ErrorMessage"=""}}, {"battery1voltage"=3.4816473, "battery2voltage"=3.4830525, "battery3voltage"=3.478369, "battery4voltage"=3.4823782, "battery5voltage"=3.4844227, "battery6voltage"=0.0, "battery7voltage"=0.0, "battery8voltage"=0.0, "battery9voltage"=0.0, "battery10voltage"=0.0, "battery11voltage"=0.0, "battery12voltage"=0.0, "battery13voltage"=0.0, "battery14voltage"=0.0, "battery15voltage"=0.0, "battery16voltage"=0.0, "battery17voltage"=0.0, "battery18voltage"=0.0, "battery19voltage"=0.0, "battery20voltage"=0.0, "battery21voltage"=0.0, "battery22voltage"=0.0, "battery23voltage"=0.0, "battery24voltage"=0.0, "ErrorOutData"={"ErrorCode"=0, "ErrorMessage"=""}}, {"battery1voltage"=3.4816477, "battery2voltage"=3.4830537, "battery3voltage"=3.4783733, "battery4voltage"=3.4823782, "battery5voltage"=3.4844193, "battery6voltage"=0.0, "battery7voltage"=0.0, "battery8voltage"=0.0, "battery9voltage"=0.0, "battery10voltage"=0.0, "battery11voltage"=0.0, "battery12voltage"=0.0, "battery13voltage"=0.0, "battery14voltage"=0.0, "battery15voltage"=0.0, "battery16voltage"=0.0, "battery17voltage"=0.0, "battery18voltage"=0.0, "battery19voltage"=0.0, "battery20voltage"=0.0, "battery21voltage"=0.0, "battery22voltage"=0.0, "battery23voltage"=0.0, "battery24voltage"=0.0, "ErrorOutData"={"ErrorCode"=0, "ErrorMessage"=""}}, {"battery1voltage"=3.481647, "battery2voltage"=3.4830585, "battery3voltage"=3.4783683, "battery4voltage"=3.4823816, "battery5voltage"=3.4844148, "battery6voltage"=0.0, "battery7voltage"=0.0, "battery8voltage"=0.0, "battery9voltage"=0.0, "battery10voltage"=0.0, "battery11voltage"=0.0, "battery12voltage"=0.0, "battery13voltage"=0.0, "battery14voltage"=0.0, "battery15voltage"=0.0, "battery16voltage"=0.0, "battery17voltage"=0.0, "battery18voltage"=0.0, "battery19voltage"=0.0, "battery20voltage"=0.0, "battery21voltage"=0.0, "battery22voltage"=0.0, "battery23voltage"=0.0, "battery24voltage"=0.0, "ErrorOutData"={"ErrorCode"=0, "ErrorMessage"=""}}, {"battery1voltage"=3.4816463, "battery2voltage"=3.4830492, "battery3voltage"=3.4783702, "battery4voltage"=3.4823797, "battery5voltage"=3.484424, "battery6voltage"=0.0, "battery7voltage"=0.0, "battery8voltage"=0.0, "battery9voltage"=0.0, "battery10voltage"=0.0, "battery11voltage"=0.0, "battery12voltage"=0.0, "battery13voltage"=0.0, "battery14voltage"=0.0, "battery15voltage"=0.0, 
